vi "Request Data JSON.vi"(8 "error in (no error)":errorcluster, 11 "GetInputKindList in":refnum<class "GetInputKindList.lvclass">) -> (0 "error out":errorcluster, 2 "Request Data JSON":string, 3 "GetInputKindList out":refnum<class "GetInputKindList.lvclass">)   [LabVIEW 2020, in "obs-websocket.lvlib" / "GetInputKindList.lvclass"]
uses:
  GetInputKindList.lvclass
  GetInputKindList.lvclass/GetInputKindList.ctl
  0bc749e0-1e2f-4b2e-909c-7af361afafae.vi
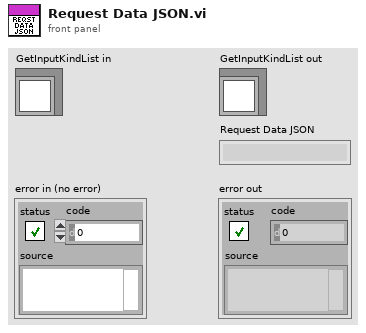
[diagram p1: front panel]
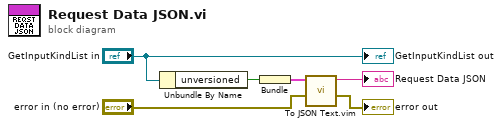
[diagram p0: block diagram]
diagram:
  n1 = Unbundle By Name("GetInputKindList in") -> ("unversioned"=w5:bool)
  n2 = Bundle("unversioned"=w5) -> (w4:cluster{"unversioned":bool})  [unwired: 1 in]
  n3 = call "To JSON Text.vim"("error in (no error)"="error in (no error)", "Anything"=w4) -> ("error out"=→"error out":errorcluster, "<JSON>"=→"Request Data JSON":string)  [unwired: 8 in]
  "GetInputKindList out" <- "GetInputKindList in"
